vi "CaptFT01-02.vi"(6 "Graph in 2":cluster{dbl[], dbl[]}, 7 "Index":i32=250, 8 "error in":errorcluster, 10 "Length 2":i32=250, 11 "ON 2":bool) -> (0 "error out":errorcluster, 2 "Values 2":cluster{dbl[], dbl[]})   [LabVIEW 2012]
uses:
  GlobalVariables/CommunicationActivity.vi
  GlobalVariables/FT02Parameters.vi
  GlobalVariables/FT01Parameters.vi
  GlobalVariables/ZeroTimeGraph.vi
  S Protocol/BrooksDLL.dll
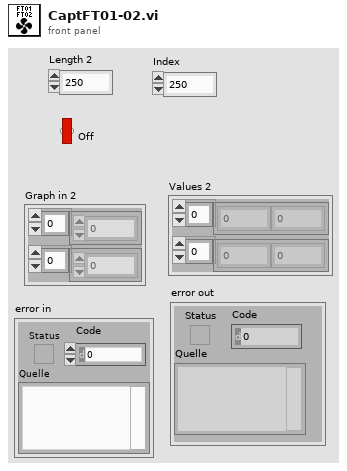
[diagram p1: front panel]
types:
  T1 = cluster{"KellerActive":bool, "GantnerActive":bool, "BrooksActive":bool}
  T2 = cluster{"KellerActive":bool, "GantnerActive":bool, bool}
  T3 = cluster{"baudrate":i32, "Port Com":i32, "Tag":u32, "FlowLimit":dbl, "IDH":u8, "IDM":u8, "IDL":u8, "IDS":u8}
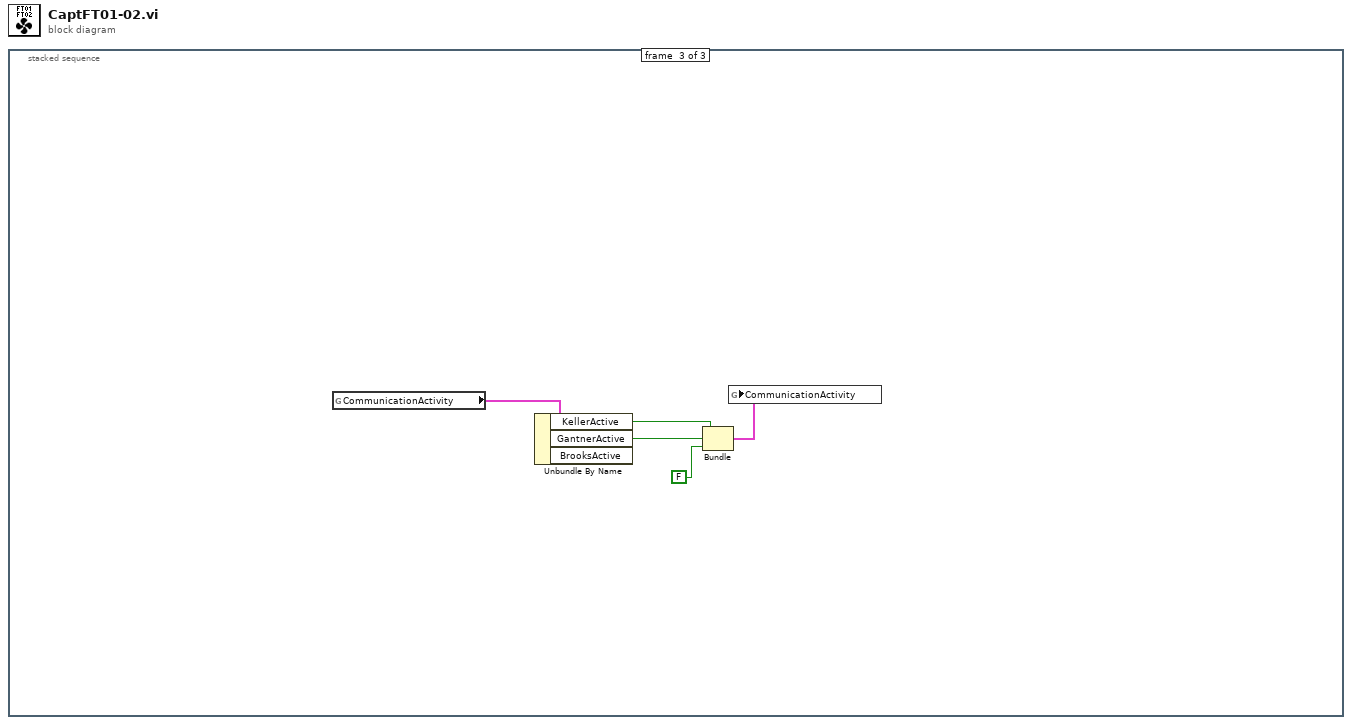
[diagram p0: block diagram]
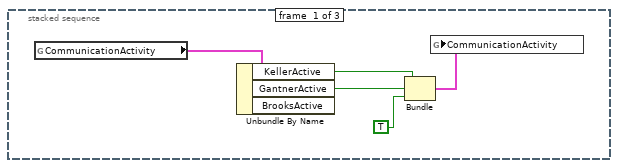
[diagram p2: hidden frame]
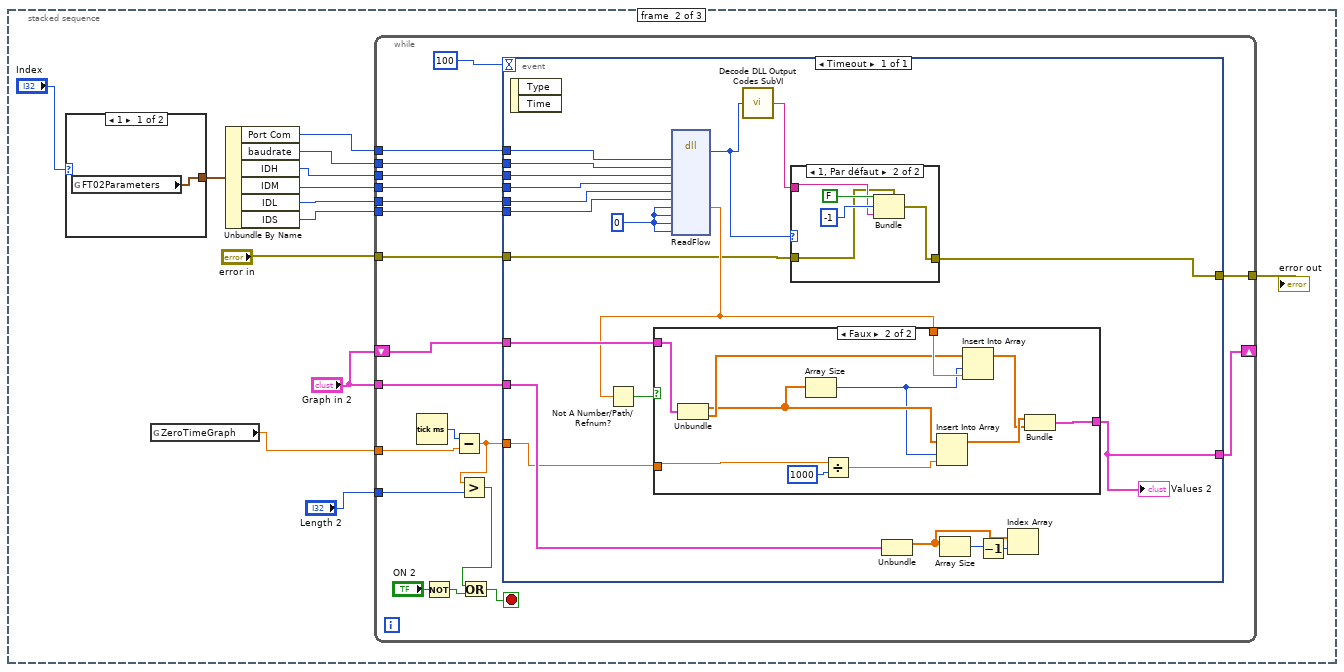
[diagram p3: hidden frame]
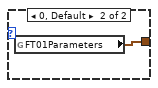
[diagram p4: hidden frame]
diagram:
  n1 = stacked-sequence {
    frame #0 {
      n2 = global read "CommunicationActivity.vi" "CommunicationActivity"() -> (w3:T1)
      n3 = Unbundle By Name(w3) -> ("KellerActive"=w2:bool, "GantnerActive"=w5:bool)  [unwired: 1 out]
      n4 = Bundle("KellerActive"=w2, "GantnerActive"=w5, TRUE) -> (w4:T2)  [unwired: 1 in]
      n5 = global write "CommunicationActivity.vi" "CommunicationActivity"(w4) -> ()
    }
    frame #1 {
      n6 = case shown="1" "Index" {
        tunnel: [w19 w20] -> w15
        frame 1 {
          n7 = global read "FT02Parameters.vi" "FT02Parameters"() -> (w19:T3)
        }
        frame 0, Default {
          n8 = global read "FT01Parameters.vi" "FT01Parameters"() -> (w20:T3)
        }
      }
      n9 = global read "ZeroTimeGraph.vi" "ZeroTimeGraph"() -> (w6:dbl)
      n10 = Unbundle By Name(w15) -> ("Port Com"=w14:i32, "baudrate"=w13:i32, "IDH"=w12:u8, "IDM"=w11:u8, "IDL"=w10:u8, "IDS"=w9:u8)
      n11 = while {
        tunnel: "error in" -> [w39]
        shift-right: [w21] -> _
        shift-left: "Graph in 2" -> [w38]
        tunnel: "Graph in 2" -> [w37]
        tunnel: w6 -> [w35]
        tunnel: "Length 2" -> [w32]
        tunnel: [w28] -> w7
        tunnel: w14 -> [w27]
        tunnel: w13 -> [w26]
        tunnel: w12 -> [w25]
        tunnel: w11 -> [w24]
        tunnel: w10 -> [w23]
        tunnel: w9 -> [w22]
        stop <- w29 stop-if-true
        n12 = Tick Count (ms)() -> (millisecond timer value=w36:u32)
        n13 = Not(x="ON 2") -> (.not. x?=w33:bool)
        n14 = Subtract(x=w36, y=w35) -> (x-y=w31:dbl)
        n15 = Greater?(x=w31, y=w32) -> (0:w30:bool)
        n16 = Or(x=w30, y=w33) -> (x .or. y?=w29:bool)
        n17 = event shown="[0] Timeout" {
          selector: _ -> [_]
          dyn-events: _ -> [_]
          timeout: 100 -> [_]
          tunnel: w39 -> [w44]
          tunnel: [w43] -> w28
          tunnel: w38 -> [w56]
          tunnel: w37 -> [w55]
          tunnel: w31 -> [w54]
          tunnel: [w53] -> w21
          tunnel: w27 -> [w51]
          tunnel: w26 -> [w50]
          tunnel: w25 -> [w49]
          tunnel: w24 -> [w46]
          tunnel: w23 -> [w47]
          tunnel: w22 -> [w48]
          event Timeout {
            w41 = 0
            n18 = event-data() -> ()  [unwired: 1 in, 2 out]
            n19 = dll-call lib="C:/Users/Sylvain/Desktop/TopPerm_20150127/drivers/Brooks/S Protocol/BrooksDLL.dll" fn="ReadFlow"("COM"=w51, "Baud"=w50, "IDH"=w49, "IDM"=w46, "IDL"=w47, "IDS"=w48, "Flow"=w41, "FlowUnit"=w41, "S1"=w41, "S2"=w41) -> (w45:i32, "Flow"=w52:sgl)  [unwired: 12 in, 2 out]
            n20 = Not A Number/Path/Refnum?(number/path/refnum=w52) -> (NaN/Path/Refnum?=w57:bool)
            n21 = case shown="Faux" w57 {
              tunnel: w54 -> [_ w78]
              tunnel: w52 -> [_ w76]
              tunnel: w56 -> [w67 w75]
              tunnel: [w67 w74] -> w53
              frame True {
              }
              frame False {
                n22 = Unbundle(w75) -> (w70:dbl[], w71:dbl[])
                n23 = Array Size(array=w70) -> (size(s)=w69:i32)
                n24 = Divide(x=w78, y=1000) -> (x/y=w68:dbl)
                n25 = Insert Into Array(array=w70, index=w69, new element=w68) -> (w73:dbl[])
                n26 = Insert Into Array(array=w71, index=w69, new element=w76) -> (w72:dbl[])
                n27 = Bundle(w73, w72) -> (w74:cluster{dbl[], dbl[]})  [unwired: 1 in]
              }
            }
            "Values 2" <- w53
            n28 = call "Decode DLL Output Codes SubVI.vi"("Numeric"=w45) -> ("Function Output Comment"=w42:string)
            n29 = case shown="1, Par défaut" w45 {
              tunnel: w44 -> [w61 w62]
              tunnel: [w61 w63] -> w43
              tunnel: w42 -> [_ w64]
              frame 0 {
              }
              frame 1, Default {
                n30 = Bundle(cluster=w62, "status"=FALSE, "code"=-1, "source"=w64) -> (w63:errorcluster)
              }
            }
            n31 = Unbundle(w55) -> (w58:dbl[])  [unwired: 1 out]
            n32 = Array Size(array=w58) -> (size(s)=w60:i32)
            n33 = Decrement(x=w60) -> (x-1=w59:i32)
            n34 = Index Array(array=w58, index=w59) -> ()  [unwired: 1 out]
          }
        }
      }
      "error out" <- w7
    }
    frame #2 {
      n35 = global read "CommunicationActivity.vi" "CommunicationActivity"() -> (w81:T1)
      n36 = Unbundle By Name(w81) -> ("KellerActive"=w80:bool, "GantnerActive"=w83:bool)  [unwired: 1 out]
      n37 = Bundle("KellerActive"=w80, "GantnerActive"=w83, FALSE) -> (w82:T2)  [unwired: 1 in]
      n38 = global write "CommunicationActivity.vi" "CommunicationActivity"(w82) -> ()
    }
  }
